vi "TorqueCurrentFOC SetControl.vi"(0 "DeviceReference":T1, 1 "Output":dbl, 2 "MaxAbsDutyCycle":dbl=1.0, 3 "Deadband":dbl, 4 "OverrideCoastDurNeutral":bool, 5 "LimitForwardMotion":bool, 6 "LimitReverseMotion":bool, 7 "error in":errorcluster, 8 "IgnoreHardwareLimits":bool, 9 "UseTimesync":bool, 18 "Update Frequency (Hz)":dbl=100.0) -> (20 "DeviceReference Out":T1, 27 "error out":errorcluster)   [LabVIEW 2023]
doc: "Request a specified motor current (field oriented control).\nThis control request will drive the motor to the requested motor (stator) current value. This leverages field oriented control (FOC), which means greater peak power than what is documented. This scales to torque based on Motor's kT constant."
uses:
  <vilib>/Rock Robotics/WPI/ThirdParty/Phoenix6/DeviceReference.ctl
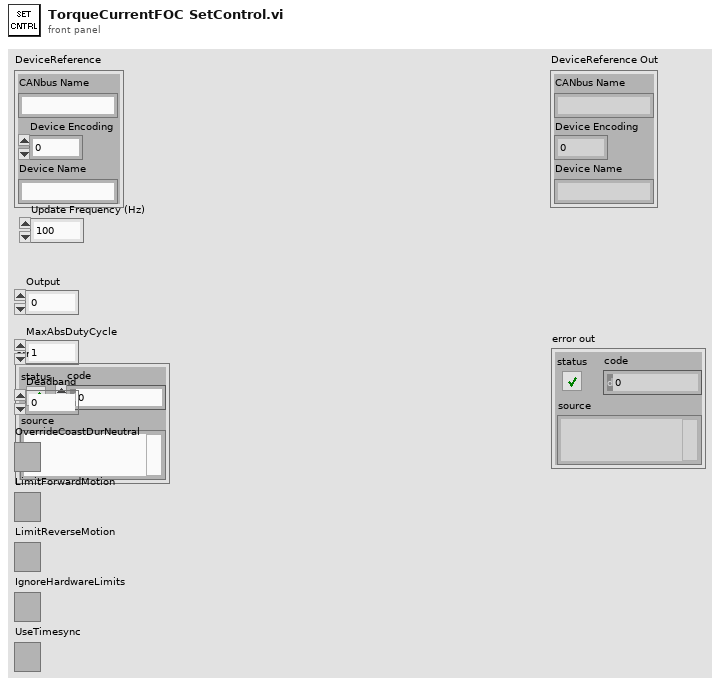
[diagram p1: front panel]
types:
  T1 = typedef "DeviceReference.ctl" = cluster{"CANbus Name":string, "Device Encoding":u32, "Device Name":string}
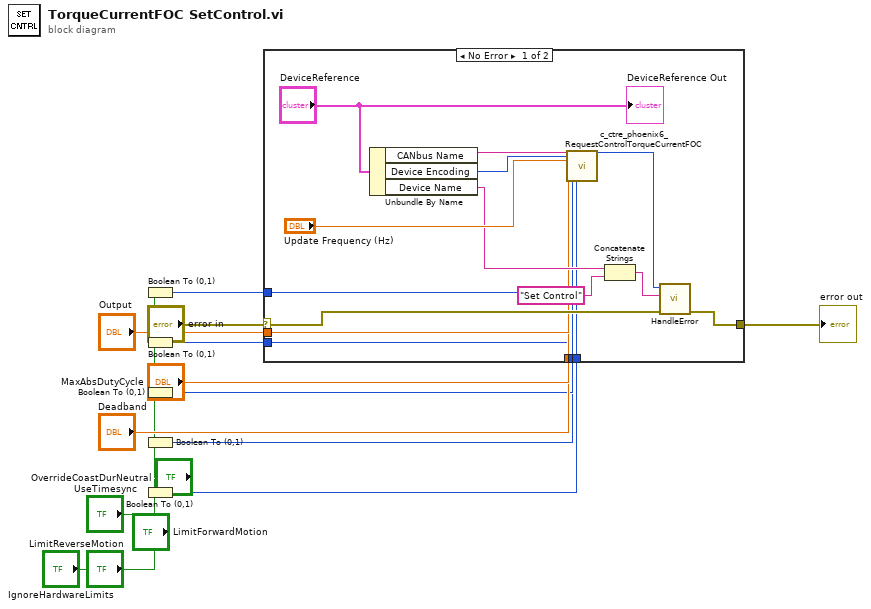
[diagram p0: block diagram]
diagram:
  n1 = Boolean To (0,1)(Boolean="OverrideCoastDurNeutral") -> (0, 1=w9:i16)
  n2 = Boolean To (0,1)(Boolean="LimitForwardMotion") -> (0, 1=w7:i16)
  n3 = Boolean To (0,1)(Boolean="LimitReverseMotion") -> (0, 1=w5:i16)
  n4 = Boolean To (0,1)(Boolean="IgnoreHardwareLimits") -> (0, 1=w3:i16)
  n5 = Boolean To (0,1)(Boolean="UseTimesync") -> (0, 1=w1:i16)
  n6 = case shown="No Error" "error in" {
    selector: "error in" -> [w28 w34]
    tunnel: [w27 w34] -> w14
    tunnel: "Output" -> [w23 _]
    tunnel: "MaxAbsDutyCycle" -> [w22 _]
    tunnel: "Deadband" -> [w21 _]
    tunnel: w9 -> [w20 _]
    tunnel: w7 -> [w19 _]
    tunnel: w5 -> [w18 _]
    tunnel: w3 -> [w17 _]
    tunnel: w1 -> [w16 _]
    frame No Error {
      n7 = Unbundle By Name("DeviceReference") -> ("CANbus Name"=w32:string, "Device Encoding"=w31:u32, "Device Name"=w26:string)
      n8 = call <vilib>:"c_ctre_phoenix6_RequestControlTorqueCurrentFOC.vi"("String 2"=w32, "Numeric 2"=w31, "Numeric 3"="Update Frequency (Hz)", "Numeric 4"=w23, "Numeric 5"=w22, "Numeric 6"=w21, "Numeric 7"=w20, "Numeric 8"=w19, "Numeric 9"=w18, "Numeric 10"=w17, "Numeric 11"=w16) -> ("Numeric"=w29:i32)  [unwired: 15 in, 1 out]
      n9 = Concatenate Strings(w26, "Set Control" ("origin")) -> (w24:string)
      n10 = call <vilib>:"HandleError.vi"("error in"=w28, "origin"=w24, "Status"=w29) -> ("error out"=w27:errorcluster)  [unwired: 8 in]
      "DeviceReference Out" <- "DeviceReference"
    }
    frame Error {
    }
  }
  "error out" <- w14
